vi "Configure Notch.vi"(5 "Bandpass Tuning Source (0: tsMeasFreq)":i32(ring) items=["tsMeasFreq", "tsAnlgGenA", "tsAnlgGenB", "tsDigGenA", "tsDigGenB", "tsSweepSrc0", "tsSweepSrc1"], 6 "Bandpass Tuning Mode (0: tmFixed)":i32(ring) items=["tmFixed", "tmTuned"], 7 "Fixed Frequency (10 Hz)":dbl=10.0, 8 "error in (no error)":errorcluster, 9 "Bandpass Filter (0: adNoNotchBP)":i32(ring) items=["adNoNotchBP", "adNotch", "adBPHW", "adBP3rdOct", "adBP6thOct", "adBP12Oct", "adBP24Oct"], 10 "Analyzer (0: A0)":i32(ring) items=["A0", "A1"], 11 "VISA resource name":refnum<visa-resource-name>) -> (0 "error out":errorcluster, 3 "VISA resource name out":refnum<visa-resource-name>)   [LabVIEW 2014, in "Stanford Research SR1.lvlib"]
doc: "Configures the attributes for the Notch."
uses:
  Stanford Research SR1.lvlib
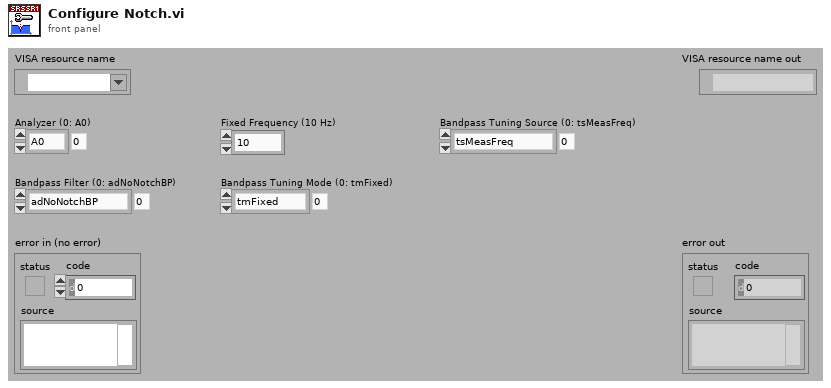
[diagram p1: front panel]
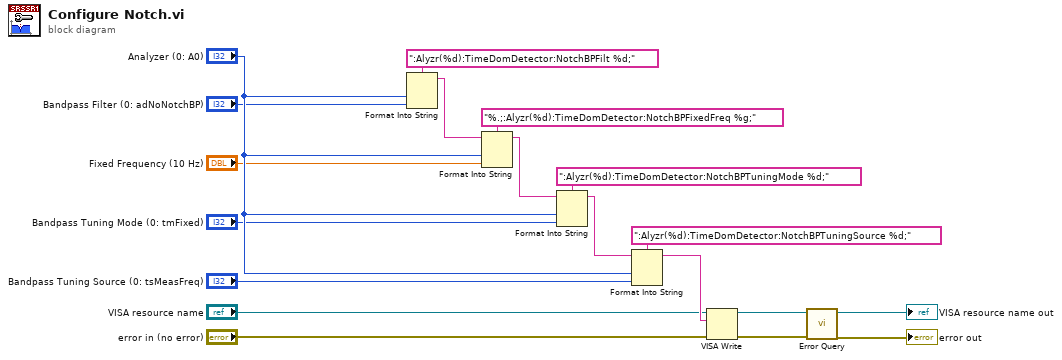
[diagram p0: block diagram]
diagram:
  n1 = Format Into String(format string=":Alyzr(%d):TimeDomDetector:NotchBPFilt %d;", "Analyzer (0: A0)", "Bandpass Filter (0: adNoNotchBP)") -> (resulting string=w18:string)  [unwired: 2 in, 1 out]
  n2 = Format Into String(format string="%.;:Alyzr(%d):TimeDomDetector:NotchBPFixedFreq %g;", initial string=w18, "Analyzer (0: A0)", "Fixed Frequency (10 Hz)") -> (resulting string=w16:string)  [unwired: 1 in, 1 out]
  n3 = Format Into String(format string=":Alyzr(%d):TimeDomDetector:NotchBPTuningMode %d;", initial string=w16, "Analyzer (0: A0)", "Bandpass Tuning Mode (0: tmFixed)") -> (resulting string=w14:string)  [unwired: 1 in, 1 out]
  n4 = Format Into String(format string=":Alyzr(%d):TimeDomDetector:NotchBPTuningSource %d;", initial string=w14, "Analyzer (0: A0)", "Bandpass Tuning Source (0: tsMeasFreq)") -> (resulting string=w12:string)  [unwired: 1 in, 1 out]
  n5 = VISA Write(VISA resource name="VISA resource name", write buffer=w12, error in (no error)="error in (no error)") -> (VISA resource name out=w9:refnum<visa-resource-name>, error out=w8:errorcluster)  [unwired: 1 out]
  n6 = call "Error Query.vi"("error in (no error)"=w8, "VISA resource name"=w9) -> ("error out"=→"error out":errorcluster, "VISA resource name out"=→"VISA resource name out":refnum<visa-resource-name>)  [unwired: 6 in, 2 out]
